vi "tkrsa6100 Config Spectrum Trace.vi"(0 "VISA Resource Name":refnum<visa-resource-name>, 1 "Trace Function\n(NORMAL)":T2(ring), 2 "Left Operand\n(TRACE 1)":enum16{"TRACE 1", "TRACE 2", "TRACE 3", "SGRAM"}(ring), 3 "Ave Count (10)":i32=10 min=2 max=10000 step=1, 5 "Set/Read\nTrace Settings (SET)":enum16{"SET", "READ"}(ring), 7 "Trace Setting\n(TRACE FUNCTION)":T3(ring), 9 "Trace # (1)":enum16{"1", "2", "3", "MATH", "SGRAM"}(ring), 11 "error in (no error)":errorcluster {"code" format="%#.0f"}, 12 "Trace Detection\n(+PEAK)":T1(ring), 13 "Right Operand\n(TRACE 1)":enum16{"TRACE 1", "TRACE 2", "TRACE 3", "SGRAM"}(ring)) -> (4 "dup VISA Resource Name":refnum<visa-resource-name>, 6 "Trace Setting\nResponse String":string, 15 "error out":errorcluster {"code" format="%#.0f"})   [LabVIEW 2020, in "Library Instrument & Equipement.lvlib" / "Library Spectrum Analyser.lvlib"]
doc: "Prerequisites for use:\n \nThis VI is valid in the Spectrum measurement view of the General Signal Viewing measurement group.\n\nThis VI controls the following functions.\nSets/reads the spectrum trace function\nSets/reads the spectrum trace detection\nSets/reads the currently selected trace\nSets/reads whether specific spectrum traces are shown or hidden\nSets/reads whether specific spectrum traces are active or frozen\nSets/reads the average count for the average trace function\nClears the trace\nSets/reads the left and right operand for the math trace function\n\nerror in (no error) is checked by tkrsa6100 Write/Read wError Query.vi for any pending errors.\n\nIf error in status is ERROR:\n\nerror in (no error) and VISA Resource Name are passed straight through to error out and dup VISA Resource Name of the Write/Read Drivers and returned to the calling function. No commands are processed.\n\nIf error in status is NO ERROR:\n\nBy passing SET to Set/Read Trace Settings (SET) the following parameters can be written. Pass the following values to Trace Settings (TRACE FUNCTION). Additional parameters to be passed are specified with each function.\n\nOne command/query is executed per VI call.\n\nTRACE FUNCTION \nSets whether the selected trace function is Normal, Average, Max Hold, or Min Hold. Pass the desired trace to enumerated control Trace # (1) and the desired function to enumerated control Trace Function (Normal). Trace functions are only valid for traces 1, 2, and 3. They are invalid for Math Trace and Spectrogram Trace (SGRAM).\n\nAVERAGE,+PEAK,-PEAK, +/-PEAK, SAMPLE, CISPR AVERAGE, CISPR PEAK , CISPR QPK, AVGLog\n\nTRACE DETECTION\nSets whether the selected trace is detected in AVERAGE,+PEAK,-PEAK, +/-PEAK, SAMPLE, CISPR AVERAGE, CISPR PEAK , CISPR QPK or AVG Log. Pass the desired trace to enumerated control Trace # (1) and the desired detection mode to enumerated control\n\nSELECT TRACE\nMakes the specified trace the \"selected\" trace (trace number that appears in the upper left corner of the display). Pass the desired trace to enumerated control Trace # (1). SGRAM trace is only valid if the Spectrogram and Spectrum measurements are both running.\n\nTRACE ON\nTRACE OFF\nShows or hides the selected trace. Pass the desired trace to enumerated control Trace # (1).\n\nFREEZE ON\nFREEZE OFF\nFreezes or allows updating of the selected trace. Pass the desired trace to enumerated control Trace # (1).\n\nAVERAGE COUNT\nSet the count for traces in average mode. Pass the desired trace to enumerated control Trace # (1) and the desired count to numeric control Ave Count (10). Average Count is only valid for traces 1, 2, and 3. It is invalid for Math Trace and Spectrogram Trace (SGRAM).\n\nCLEAR AVE/MAX/MIN (SET)\nSet Only\nClears the accumulators for traces using the Average, Max Hold, and Min Hold functions. Pass the desired trace to enumerated control Trace # (1). This function is only valid for traces 1, 2, and 3. It is invalid for Math Trace and Spectrogram Trace (SGRAM).\n\nCLEAR TRACES (SET)\nSet Only\nResets the trace for a new acquisition. Pass the desired trace to enumerated control Trace # (1). This function is only valid for traces 1, 2, and 3. It is invalid for Math Trace and Spectrogram Trace (SGRAM).\n\nLEFT OPERAND\nSets the trace to use as the left operand in the Math Trace. Pass the desired trace to use as the left operand to enumerated control Left Operand (TRACE 1). It is NOT necessary to pass a trace # to enumerated control Trace # (1), the driver is hardwired to use Trace 4 (Math Trace).\n\nRIGHT OPERAND\nSets the trace to use as the right operand in the Math Trace. Pass the desired trace to use as the right operand to enumerated control Right Operand (TRACE 1). It is NOT necessary to pass a trace # to enumerated control Trace # (1), the driver is hardwired to use Trace 4 (Math Trace).\n\nThe following parameters can be read by passing READ to enumerated control Set/Read Trace Settings (SET). Pass the following values to Trace Settings (TRACE FUNCTION). The current values are returned in string indicator Trace Settings Response String.\n\nTRACE FUNCTION\nReturns the function for the selected trace. Pass the desired trace to enumerated control Trace # (1). Trace Function is only valid for traces 1, 2, and 3. It is invalid for Math Trace and Spectrogram Trace (SGRAM).\n\n\nValid Return Values:\nNONE (Normal)\nAVER (Average)\nMAXH (Max Hold)\nMINH (Min Hold)\n\nTRACE DETECTION\nReturns the detection mode for the selected trace. Pass the desired trace to enumerated control Trace # (1). Trace Detection is only valid for traces 1, 2, and 3. It is invalid for Math Trace and Spectrogram Trace (SGRAM).\n\nValid Return Values:\nPOS (Positive)\nNEG (Negative)\nAVER (Average)\n\nSELECT TRACE\nReturns whether the specified trace is currently selected (the selected trace is the one whose number that appears in the upper left corner of the display). Pass the desired trace to enumerated control Trace # (1).\n\nValid Return Values:\n0 (Specified Trace Not Selected)\n1 (Specified Trace Selected)\n\nTRACE ON\nTRACE OFF\nEither selection returns the state of the selected trace. Pass the desired trace to enumerated control Trace # (1).\n\nValid Return Values:\n0 (Trace Off)\n1 (Trace On)\n\nFREEZE ON\nFREEZE OFF\nEither selection returns whether the selected trace is frozen or being updated. Pass the desired trace to enumerated control Trace # (1).\n\nValid Return Values:\n0 (Trace Updating)\n1 (Trace Frozen)\n\nAVERAGE COUNT\nReturns the average count for the selected trace when in average function. Pass the desired trace to enumerated control Trace # (1). Average Count is only valid for traces 1, 2, and 3. It is invalid for Math Trace and Spectrogram Trace (SGRAM).\n\nValid Return Range: 2 to 10000\n\nLEFT OPERAND\nReturns the trace that will be used as the left operand for the Math Trace. It is NOT necessary to pass a trace # to enumerated control Trace # (1), the driver is hardwired to use Trace 4 (Math Trace).\n\nValid Return Values:\nTRACE1\nTRACE2\nTRACE3\n\nRIGHT OPERAND\nReturns the trace that will be used as the right operand for the Math Trace. It is NOT necessary to pass a trace # to enumerated control Trace # (1), the driver is hardwired to use Trace 4 (Math Trace).\n\nValid Return Values:\nTRACE1\nTRACE2\nTRACE3\n\nThe appropriate command/query string is passed to tkrsa6100 Write/Read wError Query.vi. VI Input Error Query? is set to YES by default so query SYST:ERR? is appended to the command string and any current error information is displayed in cluster Error Out. \nOn completion dup VISA Resource Name, Error Out, and Trace Setting Response String are returned to the calling function."
uses:
  Library Spectrum Analyser.lvlib
panel:
  # "RSA6100 Configure Spectrum Trace Driver"
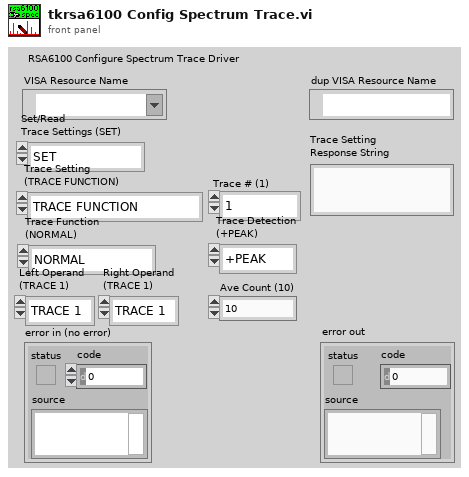
[diagram p1: front panel]
types:
  T1 = enum16{"+PEAK", "-PEAK", "AVERAGE", "SAMPLE", "CISPR AVG", "CISPR PK", "CISPR QPK", "AVERAGE LOG"}
  T2 = enum16{"NORMAL", "AVERAGE", "MAX HOLD", "MIN HOLD", "AVERAGE LOG"}
  T3 = enum16{"TRACE FUNCTION", "TRACE DETECTION", "SELECT TRACE", "TRACE ON", "TRACE OFF", "FREEZE ON", "FREEZE OFF", "AVERAGE COUNT", "CLEAR AVE/MAX/MIN (SET)", "CLEAR TRACES (SET)", "LEFT OPERAND", "RIGHT OPERAND"}
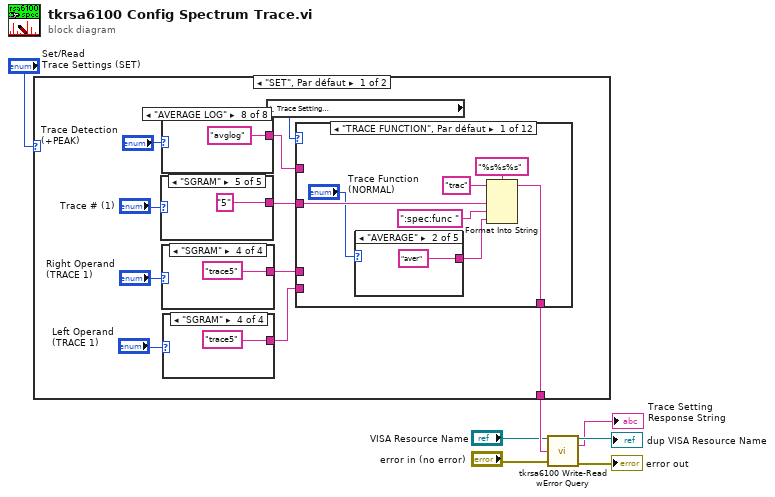
[diagram p0: block diagram]
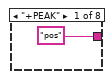
[diagram p2: hidden frame]
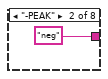
[diagram p3: hidden frame]
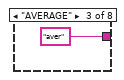
[diagram p4: hidden frame]
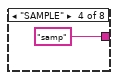
[diagram p5: hidden frame]
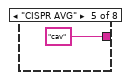
[diagram p6: hidden frame]
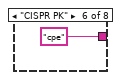
[diagram p7: hidden frame]
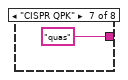
[diagram p8: hidden frame]
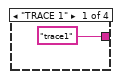
[diagram p9: hidden frame]
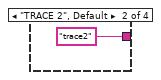
[diagram p10: hidden frame]
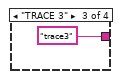
[diagram p11: hidden frame]
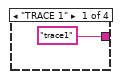
[diagram p12: hidden frame]
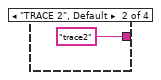
[diagram p13: hidden frame]
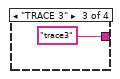
[diagram p14: hidden frame]
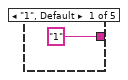
[diagram p15: hidden frame]
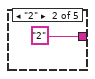
[diagram p16: hidden frame]
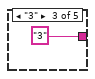
[diagram p17: hidden frame]
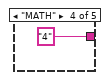
[diagram p18: hidden frame]
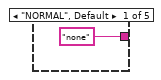
[diagram p19: hidden frame]
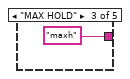
[diagram p20: hidden frame]
diagram:
  n1 = case shown="\"SET\", Par défaut" "Set/Read\nTrace Settings (SET)" {
    tunnel: [w17 w109] -> w3
    frame "SET", Default {
      n2 = case shown="\"SGRAM\"" "Trace # (1)" {
        tunnel: ["1" ("initial string") "2" ("initial string") "3" ("initial string") "4" ("initial string") "5" ("initial string")] -> w15
        frame "1", Default {
        }
        frame "2" {
        }
        frame "3" {
        }
        frame "MATH" {
        }
        frame "SGRAM" {
        }
      }
      n3 = case shown="\"AVERAGE LOG\"" "Trace Detection\n(+PEAK)" {
        tunnel: ["pos" ("initial string") "neg" ("initial string") "aver" ("initial string") "samp" ("initial string") "cav" ("initial string") "cpe" ("initial string") "quas" ("initial string") "avglog" ("initial string")] -> w8
        frame "+PEAK" {
        }
        frame "-PEAK" {
        }
        frame "AVERAGE" {
        }
        frame "SAMPLE" {
        }
        frame "CISPR AVG" {
        }
        frame "CISPR PK" {
        }
        frame "CISPR QPK" {
        }
        frame "AVERAGE LOG" {
        }
      }
      n4 = case shown="\"SGRAM\"" "Right Operand\n(TRACE 1)" {
        tunnel: ["trace1" ("initial string") "trace2" ("initial string") "trace3" ("initial string") "trace5" ("initial string")] -> w10
        frame "TRACE 1" {
        }
        frame "TRACE 2", Default {
        }
        frame "TRACE 3" {
        }
        frame "SGRAM" {
        }
      }
      n5 = case shown="\"SGRAM\"" "Left Operand\n(TRACE 1)" {
        tunnel: ["trace1" ("initial string") "trace2" ("initial string") "trace3" ("initial string") "trace5" ("initial string")] -> w11
        frame "TRACE 1" {
        }
        frame "TRACE 2", Default {
        }
        frame "TRACE 3" {
        }
        frame "SGRAM" {
        }
      }
      n6 = local read "Trace Setting\n(TRACE FUNCTION)"() -> (w14:T3)
      n7 = case shown="\"TRACE FUNCTION\", Par défaut" w14 {
        tunnel: [w43 w55 w60 w65 w70 w75 w78 w86 w91 ":spec:cle:res" ("input 2") w98 w104] -> w17
        tunnel: w15 -> [w42 w52 w57 w62 w67 w72 w77 w83 w88 _ _ _]
        tunnel: w11 -> [_ _ _ _ _ _ _ _ _ _ w95 _]
        tunnel: w10 -> [_ _ _ _ _ _ _ _ _ _ _ w101]
        tunnel: w8 -> [_ w51 _ _ _ _ _ _ _ _ _ _]
        frame "TRACE FUNCTION", Default {
          n8 = case shown="\"AVERAGE\"" "Trace Function\n(NORMAL)" {
            tunnel: ["none" ("initial string") "aver" ("initial string") "maxh" ("initial string") "minh" ("initial string") "avglog" ("initial string")] -> w39
            frame "NORMAL", Default {
            }
            frame "AVERAGE" {
            }
            frame "MAX HOLD" {
            }
            frame "MIN HOLD" {
            }
            frame "AVERAGE LOG" {
            }
          }
          n9 = Format Into String(format string="%s%s%s", initial string="trac" ("input 1"), w42, ":spec:func " ("input 2"), w39) -> (resulting string=w43:string)  [unwired: 1 in, 1 out]
        }
        frame "TRACE DETECTION" {
          n10 = Format Into String(format string="%s%s%s", initial string="trac", w52, ":spec:det " ("input 2"), w51) -> (resulting string=w55:string)  [unwired: 1 in, 1 out]
        }
        frame "SELECT TRACE" {
          n11 = Format Into String(format string="%s%s", initial string="trac", w57, ":spec:select" ("input 2")) -> (resulting string=w60:string)  [unwired: 1 in, 1 out]
        }
        frame "TRACE ON" {
          n12 = Format Into String(format string="%s%s", initial string="trac", w62, ":spec on" ("input 2")) -> (resulting string=w65:string)  [unwired: 1 in, 1 out]
        }
        frame "TRACE OFF" {
          n13 = Format Into String(format string="%s%s", initial string="trac", w67, ":spec off" ("input 2")) -> (resulting string=w70:string)  [unwired: 1 in, 1 out]
        }
        frame "FREEZE ON" {
          n14 = Format Into String(format string="%s%s", initial string="trac", w72, ":spec:fre on" ("input 2")) -> (resulting string=w75:string)  [unwired: 1 in, 1 out]
        }
        frame "FREEZE OFF" {
          n15 = Format Into String(format string="%s%s", initial string="trac" ("input 1"), w77, ":spec:fre off" ("input 4")) -> (resulting string=w78:string)  [unwired: 1 in, 1 out]
        }
        frame "AVERAGE COUNT" {
          n16 = Format Into String(format string="%s%s%d", initial string="trac", w83, ":spec:aver:coun " ("input 2"), "Ave Count (10)") -> (resulting string=w86:string)  [unwired: 1 in, 1 out]
        }
        frame "CLEAR AVE/MAX/MIN (SET)" {
          n17 = Format Into String(format string="%s%s", initial string="trac", w88, ":spec:aver:reset " ("input 2")) -> (resulting string=w91:string)  [unwired: 1 in, 1 out]
        }
        frame "CLEAR TRACES (SET)" {
        }
        frame "LEFT OPERAND" {
          n18 = Format Into String(format string="%s%s%s", initial string="trac", "4" ("initial string"), ":spec:left " ("input 2"), w95) -> (resulting string=w98:string)  [unwired: 1 in, 1 out]
        }
        frame "RIGHT OPERAND" {
          n19 = Format Into String(format string="%s%s%s", initial string="trac", "4" ("initial string"), ":spec:righ " ("input 2"), w101) -> (resulting string=w104:string)  [unwired: 1 in, 1 out]
        }
      }
    }
    frame "READ" {
      n20 = local read "Trace # (1)"() -> (w107:enum16{"1", "2", "3", "MATH", "SGRAM"})
      n21 = case shown="\"SGRAM\"" w107 {
        tunnel: ["1" ("initial string") "2" ("initial string") "3" ("initial string") "4" ("initial string") "5" ("initial string")] -> w106
        frame "1", Default {
        }
        frame "2" {
        }
        frame "3" {
        }
        frame "MATH" {
        }
        frame "SGRAM" {
        }
      }
      n22 = case shown="\"SELECT TRACE\"" "Trace Setting\n(TRACE FUNCTION)" {
        tunnel: [w118 w123 w128 w133 w138 w143 w148 w153 w158 w163] -> w109
        tunnel: w106 -> [w115 w120 w125 w130 w135 w140 w145 w150 _ _]
        frame "TRACE FUNCTION", Default {
          n23 = Format Into String(format string="%s%s", initial string="trac", w115, ":spec:func?" ("input 2")) -> (resulting string=w118:string)  [unwired: 1 in, 1 out]
        }
        frame "TRACE DETECTION" {
          n24 = Format Into String(format string="%s%s", initial string="trac", w120, ":spec:det?" ("input 2")) -> (resulting string=w123:string)  [unwired: 1 in, 1 out]
        }
        frame "TRACE ON" {
          n25 = Format Into String(format string="%s%s", initial string="trac", w125, ":spec?" ("input 2")) -> (resulting string=w128:string)  [unwired: 1 in, 1 out]
        }
        frame "SELECT TRACE" {
          n26 = Format Into String(format string="%s%s", initial string="trac", w130, ":spec:select?" ("input 2")) -> (resulting string=w133:string)  [unwired: 1 in, 1 out]
        }
        frame "TRACE OFF" {
          n27 = Format Into String(format string="%s%s", initial string="trac", w135, ":spec?" ("input 2")) -> (resulting string=w138:string)  [unwired: 1 in, 1 out]
        }
        frame "FREEZE ON" {
          n28 = Format Into String(format string="%s%s", initial string="trac", w140, ":spec:fre?" ("input 2")) -> (resulting string=w143:string)  [unwired: 1 in, 1 out]
        }
        frame "FREEZE OFF" {
          n29 = Format Into String(format string="%s%s", initial string="trac", w145, ":spec:fre?" ("input 2")) -> (resulting string=w148:string)  [unwired: 1 in, 1 out]
        }
        frame "AVERAGE COUNT" {
          n30 = Format Into String(format string="%s%s", initial string="trac", w150, ":spec:aver:coun?" ("input 2")) -> (resulting string=w153:string)  [unwired: 1 in, 1 out]
        }
        frame "LEFT OPERAND" {
          n31 = Format Into String(format string="%s%s", initial string="trac", "4" ("initial string"), ":spec:left?" ("input 2")) -> (resulting string=w158:string)  [unwired: 1 in, 1 out]
        }
        frame "RIGHT OPERAND" {
          n32 = Format Into String(format string="%s%s", initial string="trac", "4" ("initial string"), ":spec:righ?" ("input 2")) -> (resulting string=w163:string)  [unwired: 1 in, 1 out]
        }
      }
    }
  }
  n33 = call "tkrsa6100 Write-Read wError Query.vi"("VISA Resource Name"="VISA Resource Name", "Command (Empty String)"=w3, "error in (no error)"="error in (no error)") -> ("dup VISA Resource Name"=→"dup VISA Resource Name":refnum<visa-resource-name>, "Response"=→"Trace Setting\nResponse String":string, "error out"=→"error out":errorcluster)  [unwired: 4 in, 6 out]
